vi "Write data value reference.vi"(8 "error in (no error)":errorcluster, 10 "data value reference":refnum<data-value>, 11 "DAQVoltage in":refnum<class "DAQVoltage.lvclass">) -> (0 "error out":errorcluster, 3 "DAQVoltage out":refnum<class "DAQVoltage.lvclass">)   [LabVIEW 2025, in "DAQVoltage.lvlib" / "DAQVoltage.lvclass"]
uses:
  DAQVoltage.lvclass
  DAQVoltage.lvclass/DAQVoltage.ctl
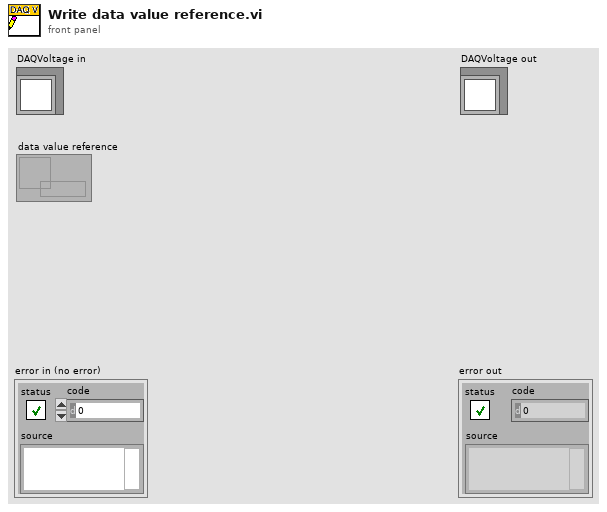
[diagram p1: front panel]
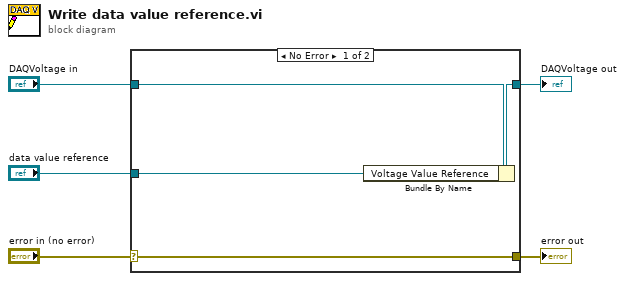
[diagram p0: block diagram]
diagram:
  n1 = case shown="No Error" "error in (no error)" {
    selector: "error in (no error)" -> [w9 w10]
    tunnel: [w9 w10] -> w4
    tunnel: [w7 w11] -> w2
    tunnel: "DAQVoltage in" -> [w8 w11]
    tunnel: "data value reference" -> [w6 _]
    frame No Error {
      n2 = Bundle By Name(cluster=w8, "Voltage Value Reference"=w6) -> (w7:refnum<class "DAQVoltage.lvclass">)
    }
    frame Error {
    }
  }
  "error out" <- w4
  "DAQVoltage out" <- w2
